vi "process.vi"(8 "error in":errorcluster, 9 "result allocation":T1, 10 "parameters":T1, 11 "module in":refnum<class "E2E Runtime (UDP).lvclass">) -> (0 "error out":errorcluster, 1 "results":T1, 2 "parameter allocation":T1, 3 "module out":refnum<class "E2E Runtime (UDP).lvclass">)   [LabVIEW 2015, in "E2E Runtime (UDP).lvclass"]
doc: "Provides an interface for information processing by a module at runtime. While this interface performs no operations, a child should provide an override which may process data in any manner necessary."
uses:
  E2E Runtime (UDP).lvclass
  <vilib>/NI/Tag Bus/table/data table.ctl
  E2E Runtime (UDP).lvclass/E2E Runtime (UDP).ctl
  <vilib>/NI/Tag Bus/table/data polymorphs/write one/write Double.vi
  <vilib>/NI/Tag Bus/table/data table.lvlib
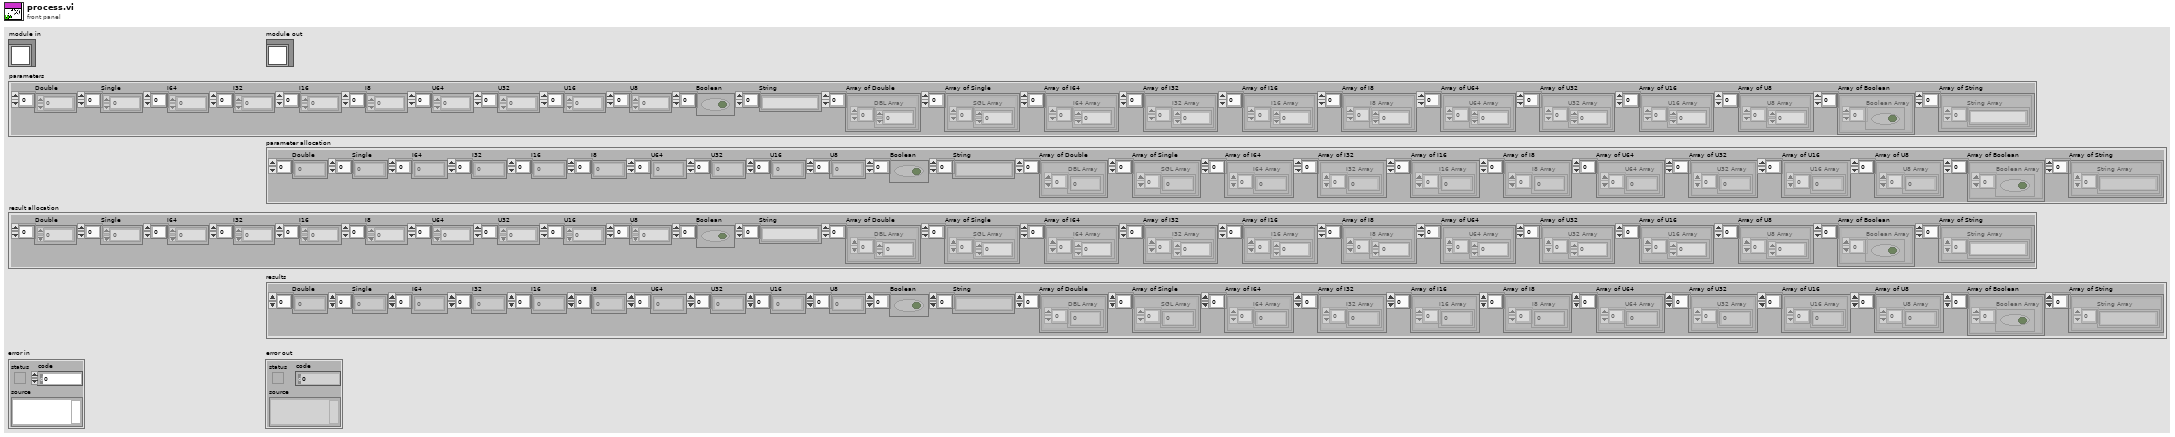
[diagram p1: front panel]
types:
  T1 = typedef "tag bus.lvlib/data table.lvlib/data table.ctl" = cluster{"Double":dbl[], "Single":sgl[], "I64":i64[], "I32":i32[], "I16":i16[], "I8":i8[], "U64":u64[], "U32":u32[], "U16":u16[], "U8":u8[], "Boolean":bool[], "String":string[], "Array of Double":cluster{"DBL Array":dbl[]}[], "Array of Single":cluster{"SGL Array":sgl[]}[], "Array of I64":cluster{"I64 Array":i64[]}[], "Array of I32":cluster{"I32 Array":i32[]}[], "Array of I16":cluster{"I16 Array":i16[]}[], "Array of I8":cluster{"I8 Array":i8[]}[], "Array of U64":cluster{"U64 Array":u64[]}[], "Array of U32":cluster{"U32 Array":u32[]}[], "Array of U16":cluster{"U16 Array":u16[]}[], "Array of U8":cluster{"U8 Array":u8[]}[], "Array of Boolean":cluster{"Boolean Array":bool[]}[], "Array of String":cluster{"String Array":string[]}[]}
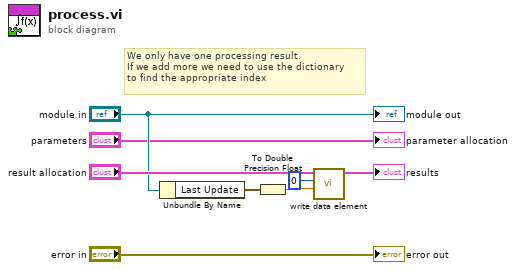
[diagram p0: block diagram]
diagram:
  # "We only have one processing result.\nIf we add more we need to use the dictionary\nto find the appropriate index"
  n1 = Unbundle By Name("module in") -> ("Last Update"=w6:timestamp)
  n2 = To Double Precision Float(number=w6) -> (double precision float=w4:dbl)
  n3 = call-poly <vilib>:"write data element.vi"("value"=w4, "index"=0, "data table in"="result allocation") -> ("data table out"=→"results":T1)  [unwired: 8 in]
  "error out" <- "error in"
  "module out" <- "module in"
  "parameter allocation" <- "parameters"
